vi "Insert Loop.vi"(4 "Loop Iterations":i32, 6 "Insertion Index":i32=-1, 7 "Parent ID":string, 8 "error in (no error)":errorcluster, 9 "Unique ID":string, 10 "Name":string, 11 "Test Executive in":refnum<class "Test Executive.lvclass">) -> (0 "error out":errorcluster, 1 "Replaced?":bool, 2 "Unique ID out":string, 3 "Test Executive out":refnum<class "Test Executive.lvclass">)   [LabVIEW 2017, in "Test Executive.lvlib" / "Test Executive.lvclass"]
uses:
  <vilib>/gpm_packages/@cs/test-executive/Source/Test Executive/TestExecutive/Test Executive.lvclass
  <vilib>/gpm_packages/@cs/test-executive/Source/Test Executive/Loop/Loop.lvclass
  <vilib>/gpm_packages/@cs/test-executive/Source/Test Executive/TestExecutive/Test Executive.lvclass/Test Executive.ctl
  152cdfc5-d1e9-4c56-99d6-cf0348d6af82.vi
  61e5cccf-d0ee-4683-84d1-07d0b43a0ba0.vi
  147e2e27-9108-4dad-9c96-1b8cc2834f97.vi
  a0e54f6b-bb11-461c-a7f2-8fa2e5b52b2c.vi
  <vilib>/gpm_packages/@cs/linked-list/Source/Linked List/ILinkedList/ILinked List.lvclass
  <vilib>/gpm_packages/@cs/linked-list/Source/Linked List/Linked List Ref/Linked List Ref.lvclass
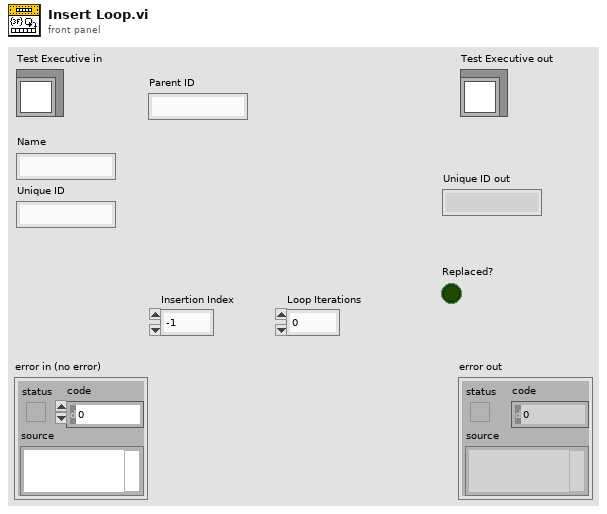
[diagram p1: front panel]
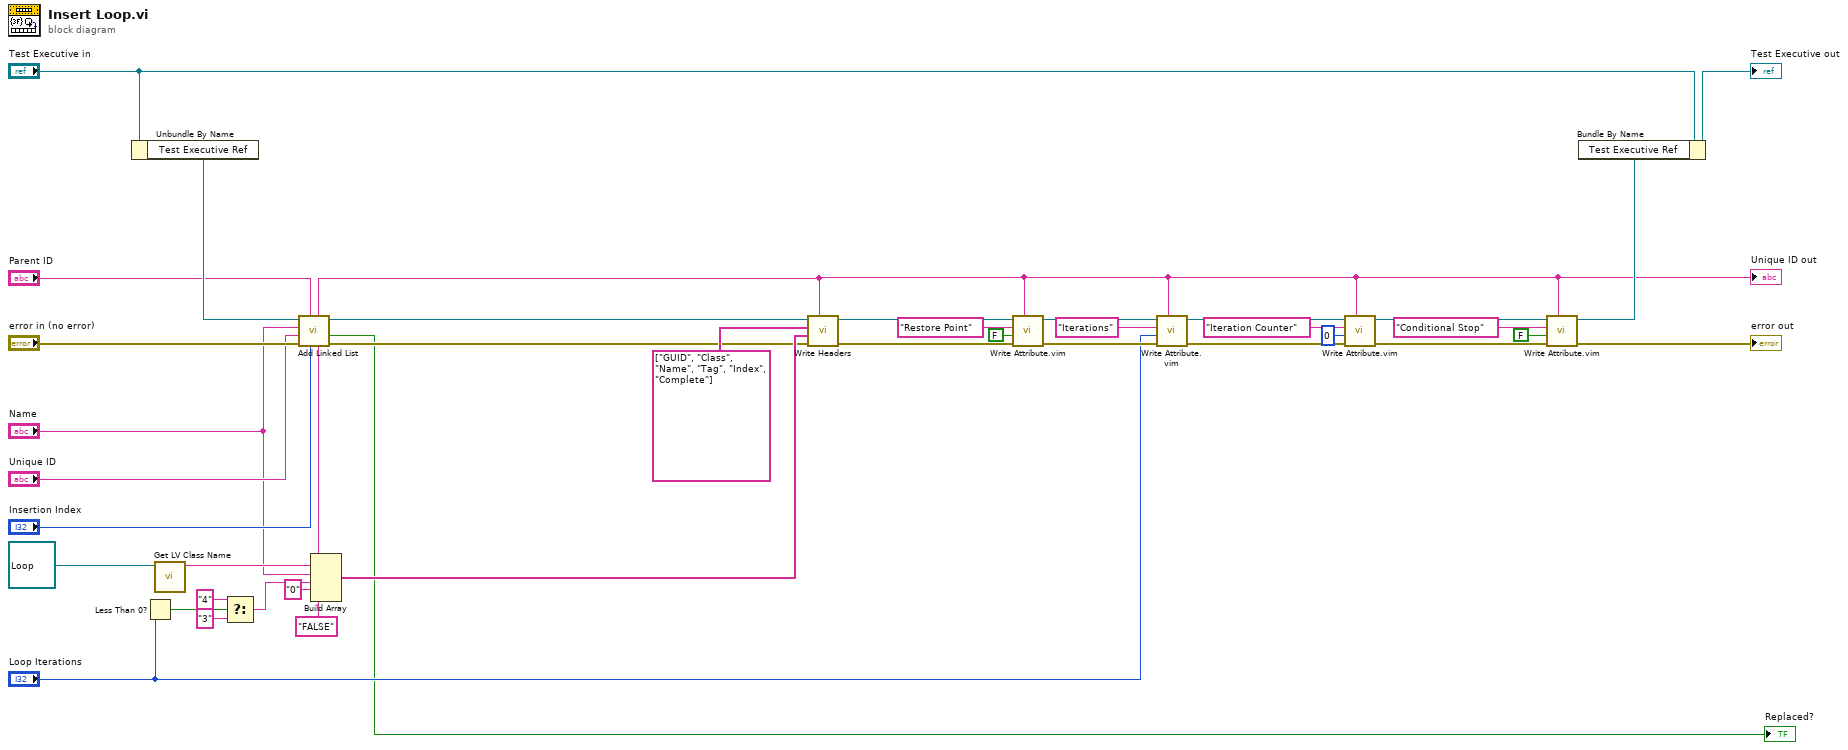
[diagram p0: block diagram]
diagram:
  n1 = Unbundle By Name("Test Executive in") -> ("Test Executive Ref"=w39:refnum<data-value>)
  n2 = Less Than 0?(x="Loop Iterations") -> (x < 0?=w24:bool)
  n3 = call <vilib>:"Get LV Class Name.vi"("object"=refnum<class "Loop.lvclass"> refnum ("Test Executive.lvlib:Loop.lvclass")) -> ("class name"=w30:string)  [unwired: 9 in, 1 out]
  n4 = Select(t="4" ("Tag"), s=w24, f="3" ("Tag")) -> (s? t:f=w21:string)
  n5 = call <vilib>:"Add Linked List.vi"("Insertion Index"="Insertion Index", "Parent ID"="Parent ID", "error in (no error)"="error in (no error)", "Linked List ID"="Unique ID", "Name"="Name", "Linked List Ref"=w39) -> ("error out"=w32:errorcluster, "Replaced?"=→"Replaced?":bool, "Linked List Ref out"=w33:refnum<data-value>, "Linked List ID out"=w2:string)  [unwired: 2 in]
  "Unique ID out" <- w2
  n6 = Build Array(w2, w30, "Name", w21, "0" ("element"), "FALSE" ("element")) -> (w34:string[])
  n7 = call <vilib>:"Write Headers.vi"("Linked List ID"=w2, "error in (no error)"=w32, "Header Values"=w34, "Header Names"=string[] ["GUID", "Class", "Name", "Tag", "Index", "Complete"], "Linked List Ref"=w33) -> ("error out"=w25:errorcluster, "Linked List Ref out"=w26:refnum<data-value>)  [unwired: 5 in]
  n8 = call "Write Attribute.vim"("Linked List ID"=w2, "error in (no error)"=w25, "Attribute"=FALSE, "Attribute Name"="Restore Point", "Linked List Ref"=w26) -> ("error out"=w14:errorcluster, "Linked List Ref out"=w17:refnum<data-value>)  [unwired: 3 in, 2 out]
  n9 = call "Write Attribute.vim"("Linked List ID"=w2, "error in (no error)"=w14, "Attribute"="Loop Iterations", "Attribute Name"="Iterations", "Linked List Ref"=w17) -> ("error out"=w13:errorcluster, "Linked List Ref out"=w16:refnum<data-value>)  [unwired: 3 in, 2 out]
  n10 = call "Write Attribute.vim"("Linked List ID"=w2, "error in (no error)"=w13, "Attribute"=0 ("Numeric"), "Attribute Name"="Iteration Counter", "Linked List Ref"=w16) -> ("error out"=w12:errorcluster, "Linked List Ref out"=w15:refnum<data-value>)  [unwired: 3 in, 2 out]
  n11 = call "Write Attribute.vim"("Linked List ID"=w2, "error in (no error)"=w12, "Attribute"=FALSE ("Boolean"), "Attribute Name"="Conditional Stop", "Linked List Ref"=w15) -> ("error out"=→"error out":errorcluster, "Linked List Ref out"=w5:refnum<data-value>)  [unwired: 3 in, 2 out]
  n12 = Bundle By Name(cluster="Test Executive in", "Test Executive Ref"=w5) -> (→"Test Executive out":refnum<class "Test Executive.lvclass">)
